vi "Unit Test.vi"() -> ()   [LabVIEW 2017]
uses:
  builds/Built/Power_Supply.lvlibp/Power Supply.lvclass
panel:
  out "mOutput":bool
  out "mCurrent":dbl
  out "mVoltage":dbl
  in  "Output":bool
  in  "Current":dbl
  in  "Voltage":dbl
  in  "stop":bool
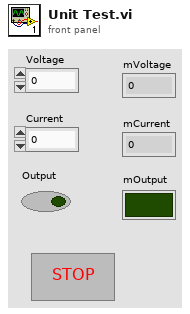
[diagram p1: front panel]
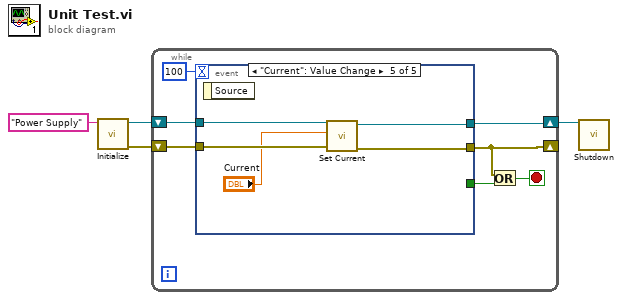
[diagram p0: block diagram]
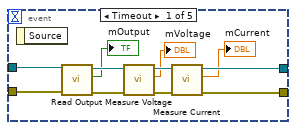
[diagram p2: hidden frame]
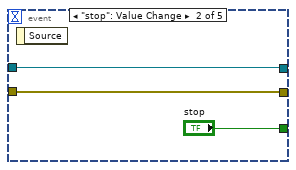
[diagram p3: hidden frame]
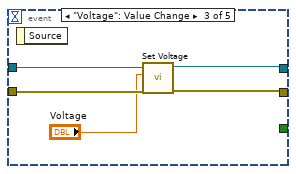
[diagram p4: hidden frame]
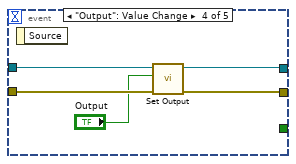
[diagram p5: hidden frame]
diagram:
  n1 = call "Initialize.vi"("Device"="Power Supply") -> ("error out"=w2:errorcluster, "Power Supply out"=w3:refnum<class "Power Supply.lvclass">)  [unwired: 9 in]
  n2 = while {
    shift-right: [w9] -> w1
    shift-left: w3 -> [w10]
    shift-right: [w6] -> _
    shift-left: w2 -> [w8]
    stop <- w11 stop-if-true
    n3 = event shown="[4] \"Current\": Value Change" {
      selector: _ -> [_ _ _ _ _]
      dyn-events: _ -> [_ _ _ _ _]
      timeout: 100 -> [_ _ _ _ _]
      tunnel: w10 -> [w22 w25 w30 w35 w40]
      tunnel: [w19 w25 w29 w32 w37] -> w9
      tunnel: w8 -> [w18 w24 w27 w34 w39]
      tunnel: [w15 w24 w28 w33 w38] -> w6
      tunnel: [_ "stop" _ _ _] -> w5
      event Timeout {
        n4 = event-data() -> ()  [unwired: 1 in, 1 out]
        n5 = call-dynamic "Read Output.vi"("error in"=w18, "Power Supply in"=w22) -> ("error out"=w17:errorcluster, "Output"=→"mOutput":bool, "Power Supply out"=w21:refnum<class "Power Supply.lvclass">)  [unwired: 7 in]
        n6 = call-dynamic "Measure Voltage.vi"("error in (no error)"=w17, "Power Supply in"=w21) -> ("error out"=w16:errorcluster, "Voltage"=→"mVoltage":dbl, "Power Supply out"=w20:refnum<class "Power Supply.lvclass">)  [unwired: 7 in]
        n7 = call-dynamic "Measure Current.vi"("error in (no error)"=w16, "Power Supply in"=w20) -> ("error out"=w15:errorcluster, "Current"=→"mCurrent":dbl, "Power Supply out"=w19:refnum<class "Power Supply.lvclass">)  [unwired: 7 in]
      }
      event "stop": Value Change {
        n8 = event-data() -> ()  [unwired: 1 in, 1 out]
      }
      event "Voltage": Value Change {
        n9 = event-data() -> ()  [unwired: 1 in, 1 out]
        n10 = call "Set Voltage.vi"("error in"=w27, "Voltage"="Voltage", "Power Supply in"=w30) -> ("error out"=w28:errorcluster, "Power Supply out"=w29:refnum<class "Power Supply.lvclass">)  [unwired: 7 in]
      }
      event "Output": Value Change {
        n11 = event-data() -> ()  [unwired: 1 in, 1 out]
        n12 = call "Set Output.vi"("error in"=w34, "Output"="Output", "Power Supply in"=w35) -> ("error out"=w33:errorcluster, "Power Supply out"=w32:refnum<class "Power Supply.lvclass">)  [unwired: 7 in]
      }
      event "Current": Value Change {
        n13 = event-data() -> ()  [unwired: 1 in, 1 out]
        n14 = call "Set Current.vi"("error in"=w39, "Current"="Current", "Power Supply in"=w40) -> ("error out"=w38:errorcluster, "Power Supply out"=w37:refnum<class "Power Supply.lvclass">)  [unwired: 7 in]
      }
    }
    n15 = Or(x=w6, y=w5) -> (x .or. y?=w11:bool)
  }
  n16 = call "Shutdown.vi"("Power Supply in"=w1) -> ()  [unwired: 9 in, 2 out]
